vi "file.IsValid.vi"(8 "error in (no error)":errorcluster, 11 "path":path) -> (0 "error out":errorcluster, 2 "valid file/folder?":bool, 3 "dup path":path)   [LabVIEW 2020]
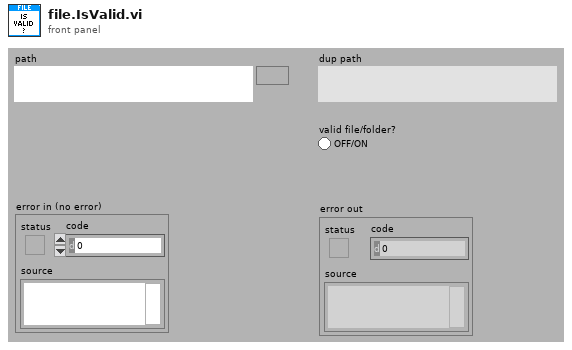
[diagram p1: front panel]
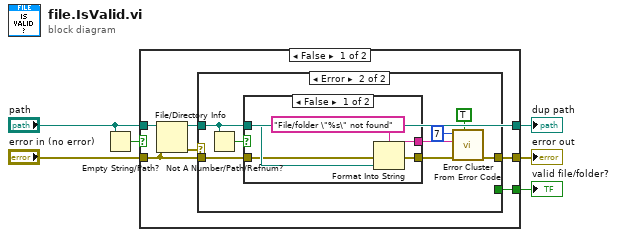
[diagram p0: block diagram]
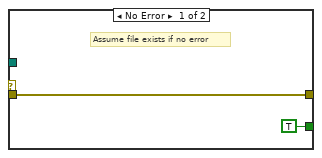
[diagram p2: hidden frame]
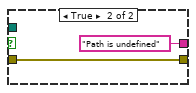
[diagram p3: hidden frame]
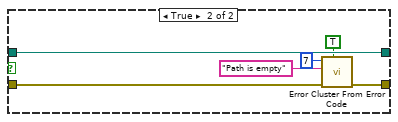
[diagram p4: hidden frame]
diagram:
  n1 = Empty String/Path?(string/path="path") -> (empty?=w1:bool)
  n2 = case shown="False" w1 {
    tunnel: "error in (no error)" -> [w7 w30]
    tunnel: "path" -> [w12 w35]
    tunnel: [w11 w35] -> w4
    tunnel: [w10 w31] -> w3
    tunnel: [w9 _] -> w2
    frame False {
      n3 = File/Directory Info(path=w12, error in=w7) -> (path out=w11:path, error out=w8:errorcluster)  [unwired: 5 out]
      n4 = case shown="Error" w8 {
        tunnel: w11 -> [_ w15]
        tunnel: [w14 w18] -> w10
        tunnel: [TRUE _] -> w9
        tunnel: w7 -> [w14 w17]
        frame No Error {
          # "Assume file exists if no error"
        }
        frame Error {
          n5 = Not A Number/Path/Refnum?(number/path/refnum=w15) -> (NaN/Path/Refnum?=w16:bool)
          n6 = case shown="False" w16 {
            tunnel: [w27 "Path is undefined"] -> w22
            tunnel: [w25 w29] -> w19
            tunnel: w15 -> [w24 _]
            tunnel: w17 -> [w23 w29]
            frame False {
              n7 = Format Into String(format string="File/folder \"%s\" not found", error in=w23, w24) -> (resulting string=w27:string, error out=w25:errorcluster)  [unwired: 1 in]
            }
            frame True {
            }
          }
          n8 = call <vilib>:"Error Cluster From Error Code.vi"("show call chain? (False)"=TRUE, "error in (no error)"=w19, "error message (\"\")"=w22, "error code (0)"=7) -> ("error out"=w18:errorcluster)  [unwired: 5 in]
        }
      }
    }
    frame True {
      n9 = call <vilib>:"Error Cluster From Error Code.vi"("show call chain? (False)"=TRUE, "error in (no error)"=w30, "error message (\"\")"="Path is empty" ("format string"), "error code (0)"=7) -> ("error out"=w31:errorcluster)  [unwired: 5 in]
    }
  }
  "valid file/folder?" <- w2
  "dup path" <- w4
  "error out" <- w3
